vi "LinearSystem_GetAElement.vi"(9 "Column":i32, 10 "Row":i32, 11 "Linearsystem":T1) -> (3 "A Element Value":dbl)   [LabVIEW 2019, in "Trajectory_Library.lvlib"]
doc: "Creates a new LINEAR SYSTEM data cluster with the specified values. \n\n\nInputs: \n - XXX -- XXX.\n\nOutputs:\n - XXX -- XXX."
uses:
  Trajectory_Library.lvlib
  LINEAR_SYSTEM.ctl
  <vilib>/Analysis/Matrix/Datatypes/RealMatrix.ctl
  <vilib>/Analysis/Matrix/NI_Matrix.lvlib
panel:
  # "<States,States>"
  # "<States,Inputs>"
  # "<Outputs,States>"
  # "<Outputs,Inputs>"
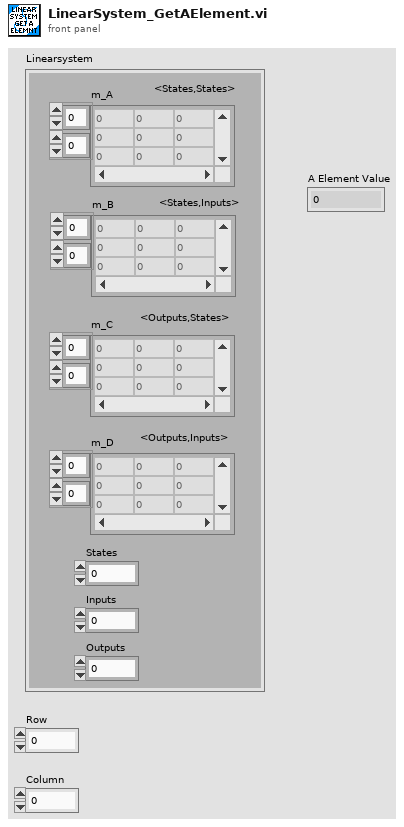
[diagram p1: front panel]
types:
  T1 = typedef "Trajectory_Library.lvlib/LINEAR_SYSTEM.ctl" = cluster{"m_A":T2, "m_B":T2, "m_C":T2, "m_D":T2, "States":i32, "Inputs":i32, "Outputs":i32}
  T2 = typedef "NI_Matrix.lvlib/RealMatrix.ctl" = dbl[][]
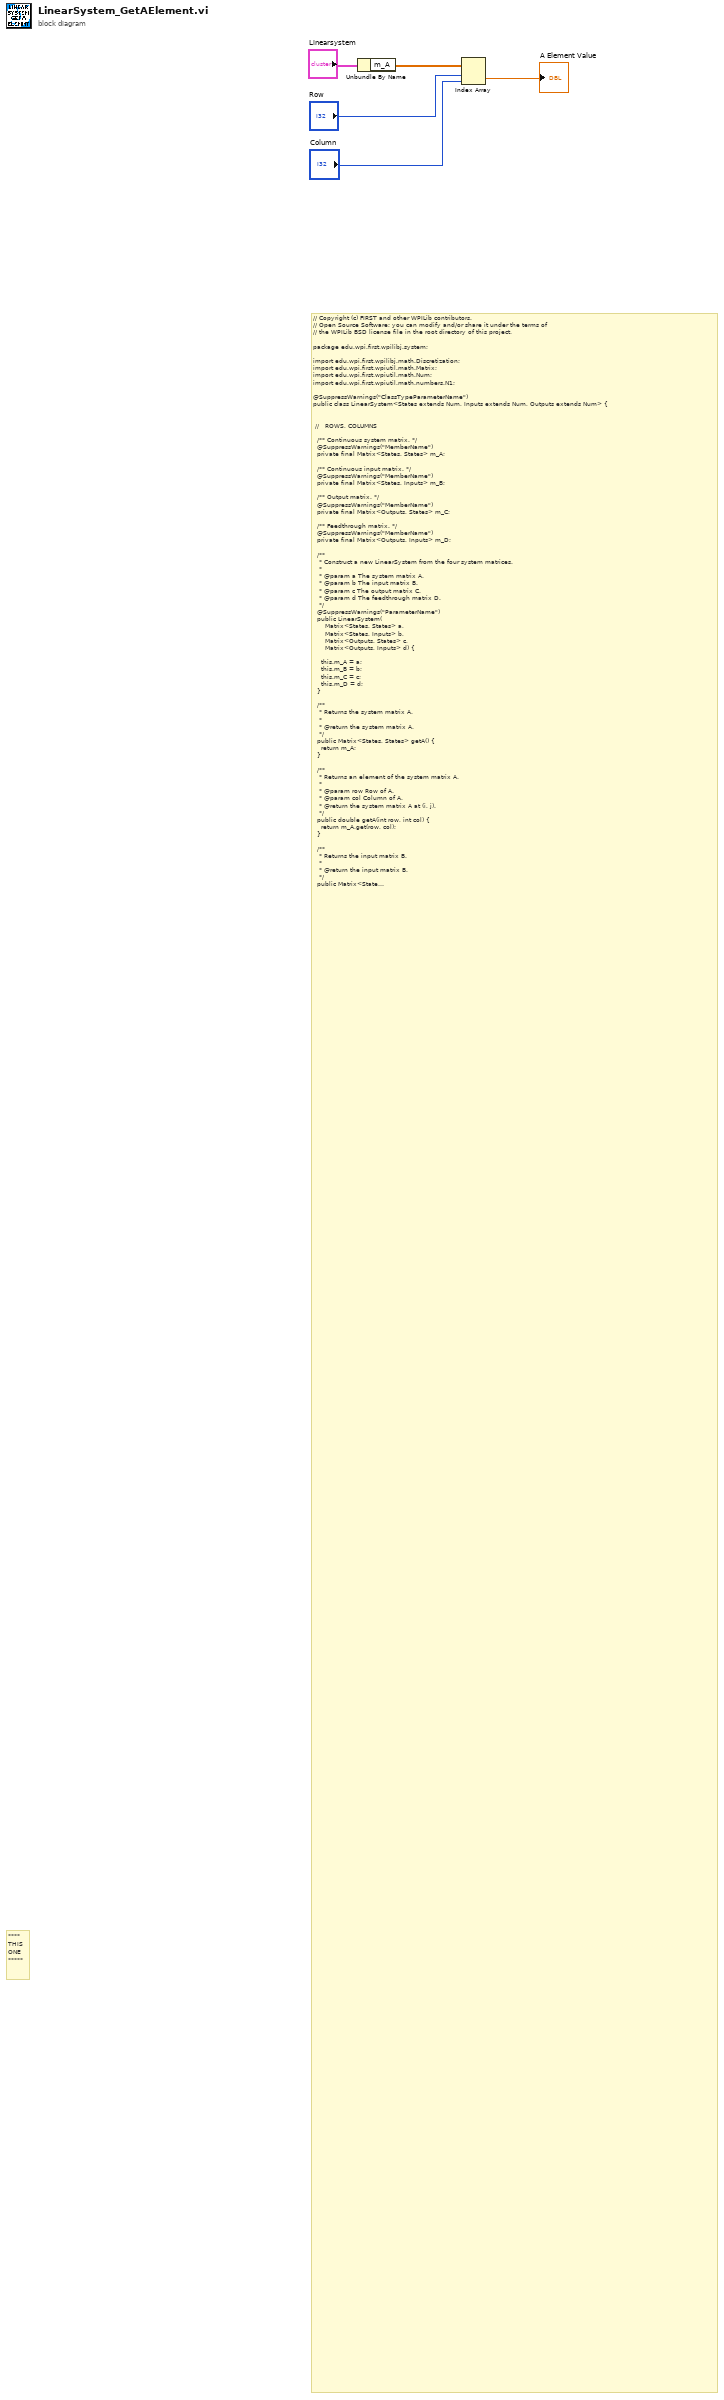
[diagram p0: block diagram]
diagram:
  # "// Copyright (c) FIRST and other WPILib contributors.\n// Open Source Software; you can modify and/or share it under the terms of\n// the WPILib BSD license file in the root directory of this project.\n\npackage edu.wpi.first.wpilibj.system;\n\nimport edu.wpi.first.wpilibj.math.Discretization;\nimport edu.wpi.first.wpiutil.math.Matrix;\nimport edu.wpi.first.wpiutil.math.Num;\nimport edu.wpi.first.wpiutil.math.numbers.N1;\n\n@SuppressWarnings(\"ClassTypeParameterName\")\npublic class LinearSystem<States extends Num, Inputs extends Num, Outputs extends Num> {\n\n\n\t//   ROWS, COLUMNS\n\n  /** Continuous system matrix. */\n  @SuppressWarnings(\"MemberName\")\n  private final Matrix<States, States> m_A;\n\n  /** Continuous input matrix. */\n  @SuppressWarnings(\"MemberName\")\n  private final Matrix<States, Inputs> m_B;\n\n  /** Output matrix. */\n  @SuppressWarnings(\"MemberName\")\n  private final Matrix<Outputs, States> m_C;\n\n  /** Feedthrough matrix. */\n  @SuppressWarnings(\"MemberName\")\n  private final Matrix<Outputs, Inputs> m_D;\n\n  /**\n   * Construct a new LinearSystem from the four system matrices.\n   *\n   * @param a The system matrix A.\n   * @param b The input matrix B.\n   * @param c The output matrix C.\n   * @param d The feedthrough matrix D.\n   */\n  @SuppressWarnings(\"ParameterName\")\n  public LinearSystem(\n      Matrix<States, States> a,\n      Matrix<States, Inputs> b,\n      Matrix<Outputs, States> c,\n      Matrix<Outputs, Inputs> d) {\n\n    this.m_A = a;\n    this.m_B = b;\n    this.m_C = c;\n    this.m_D = d;\n  }\n\n  /**\n   * Returns the system matrix A.\n   *\n   * @return the system matrix A.\n   */\n  public Matrix<States, States> getA() {\n    return m_A;\n  }\n\n  /**\n   * Returns an element of the system matrix A.\n   *\n   * @param row Row of A.\n   * @param col Column of A.\n   * @return the system matrix A at (i, j).\n   */\n  public double getA(int row, int col) {\n    return m_A.get(row, col);\n  }\n\n  /**\n   * Returns the input matrix B.\n   *\n   * @return the input matrix B.\n   */\n  public Matrix<States, Inputs> getB() {\n    return m_B;\n  }\n\n  /**\n   * Returns an element of the input matrix B.\n   *\n   * @param row Row of B.\n   * @param col Column of B.\n   * @return The value of the input matrix B at (i, j).\n   */\n  public double getB(int row, int col) {\n    return m_B.get(row, col);\n  }\n\n  /**\n   * Returns the output matrix C.\n   *\n   * @return Output matrix C.\n   */\n  public Matrix<Outputs, States> getC() {\n    return m_C;\n  }\n\n  /**\n   * Returns an element of the output matrix C.\n   *\n   * @param row Row of C.\n   * @param col Column of C.\n   * @return the double value of C at the given position.\n   */\n  public double getC(int row, int col) {\n    return m_C.get(row, col);\n  }\n\n  /**\n   * Returns the feedthrough matrix D.\n   *\n   * @return the feedthrough matrix D.\n   */\n  public Matrix<Outputs, Inputs> getD() {\n    return m_D;\n  }\n\n  /**\n   * Returns an element of the feedthrough matrix D.\n   *\n   * @param row Row of D.\n   * @param col Column of D.\n   * @return The feedthrough matrix D at (i, j).\n   */\n  public double getD(int row, int col) {\n    return m_D.get(row, col);\n  }\n\n  /**\n   * Computes the new x given the old x and the control input.\n   *\n   * <p>This is used by state observers directly to run updates based on state estimate.\n   *\n   * @param x The current state.\n   * @param clampedU The control input.\n   * @param dtSeconds Timestep for model update.\n   * @return the updated x.\n   */\n  @SuppressWarnings(\"ParameterName\")\n  public Matrix<States, N1> calculateX(\n      Matrix<States, N1> x, Matrix<Inputs, N1> clampedU, double dtSeconds) {\n    var discABpair = Discretization.discretizeAB(m_A, m_B, dtSeconds);\n\n    return (discABpair.getFirst().times(x)).plus(discABpair.getSecond().times(clampedU));\n  }\n\n  /**\n   * Computes the new y given the control input.\n   *\n   * <p>This is used by state observers directly to run updates based on state estimate.\n   *\n   * @param x The current state.\n   * @param clampedU The control input.\n   * @return the updated output matrix Y.\n   */\n  @SuppressWarnings(\"ParameterName\")\n  public Matrix<Outputs, N1> calculateY(Matrix<States, N1> x, Matrix<Inputs, N1> clampedU) {\n    return m_C.times(x).plus(m_D.times(clampedU));\n  }\n\n  @Override\n  public String toString() {\n    return String.format(\n        \"Linear System: A\\n%s\\n\\nB:\\n%s\\n\\nC:\\n%s\\n\\nD:\\n%s\\n\",\n        m_A.toString(), m_B.toString(), m_C.toString(), m_D.toString());\n  }\n}"
  # "****\nTHIS\nONE\n*****"
  n1 = Unbundle By Name("Linearsystem") -> ("m_A"=w2:T2)
  n2 = Index Array(array=w2, index (row)="Row", index (col)="Column") -> (element=→"A Element Value":dbl)
